vi "PC-2.vi"(4 "Ci-1":bool[](array[boolean]), 5 "Di-1":bool[](array[boolean]), 7 "n":i32) -> (0 "Ci":bool[](array[boolean]), 1 "Di":bool[](array[boolean]), 2 "SubKeyi":bool[](array[boolean]))   [LabVIEW 2013]
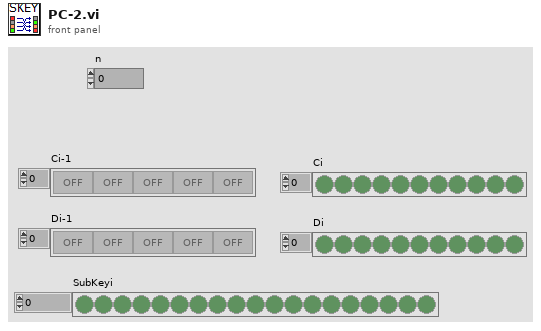
[diagram p1: front panel]
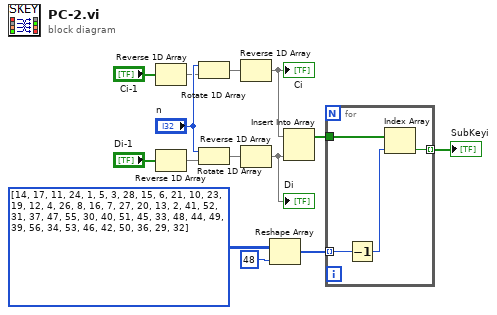
[diagram p0: block diagram]
diagram:
  n1 = Reverse 1D Array(array="Ci-1") -> (reversed array=w5:bool[])
  n2 = Reverse 1D Array(array="Di-1") -> (reversed array=w10:bool[])
  n3 = Rotate 1D Array(1:w5, 2:"n") -> (0:w11:bool[])
  n4 = Rotate 1D Array(1:w10, 2:"n") -> (0:w9:bool[])
  n5 = Reverse 1D Array(array=w11) -> (reversed array=w2:bool[])
  "Ci" <- w2
  n6 = Reverse 1D Array(array=w9) -> (reversed array=w1:bool[])
  "Di" <- w1
  n7 = Reshape Array(u8[][] [[14, 17, 11, 24, 1, 5, 3, 28], [15, 6, 21, 10, 23, 19, 12, 4], [26, 8, 16, 7, 27, 20, 13, 2], [41, 52, 31, 37, 47, 55, 30, 40], [51, 45, 33, 48, 44, 49, 39, 56], [34, 53, 46, 42, 50, 36, 29, 32]], 48 ("dimension size")) -> (w13:u8[])
  n8 = Insert Into Array(array=w2, new element=w1) -> (w8:bool[])  [unwired: 1 in]
  n9 = for {
    tunnel: w8 -> [w17]
    tunnel: w13 -> [w18] mode=indexing
    tunnel: [w15] -> w7 mode=indexing
    n10 = Decrement(x=w18) -> (x-1=w16:u8)
    n11 = Index Array(array=w17, index=w16) -> (element=w15:bool)
  }
  "SubKeyi" <- w7
